vi "Add Device.vi"(8 "error in (no error)":errorcluster, 10 "Device":refnum<class "Hardware.lvclass">, 11 "Controller in":refnum<class "Controller.lvclass">) -> (0 "error out":errorcluster, 3 "Controller out":refnum<class "Controller.lvclass">)   [LabVIEW 2016, in "Controller Actor.lvlib" / "Controller.lvclass"]
uses:
  <userlib>/Common Components/Controller/Controller.lvclass
  C:/Program Files (x86)/National Instruments/LabVIEW 2016/vi.lib/ActorFramework/Actor/Actor.lvclass
  <userlib>/Common Components/Hardware/Abstract Hardware/Hardware.lvclass
  <userlib>/Common Components/Controller/Controller.lvclass/Controller.ctl
  <vilib>/ActorFramework/Actor/Actor.lvclass/Actor.ctl
  <vilib>/ActorFramework/Message Enqueuer/Message Enqueuer.lvclass/Message Enqueuer.ctl
  <vilib>/ActorFramework/Message Enqueuer/Init from Existing Queue.vi
  <vilib>/ActorFramework/Message Enqueuer/Message Enqueuer.lvclass
  <userlib>/Common Components/Controller/Messages/Log Status/Log Status.lvclass
  <vilib>/ActorFramework/Actor/Actor.lvclass
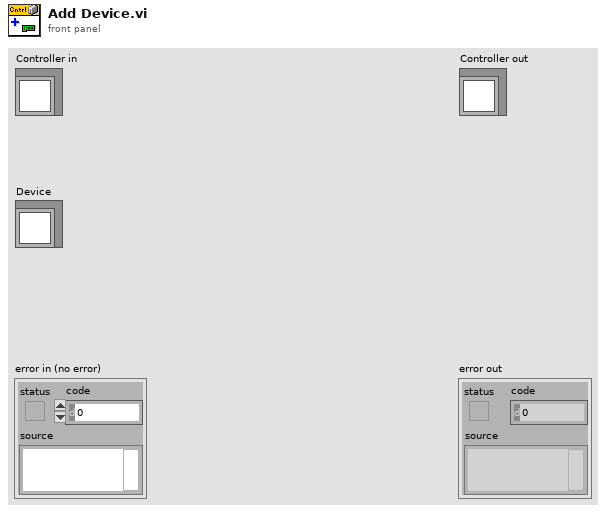
[diagram p1: front panel]
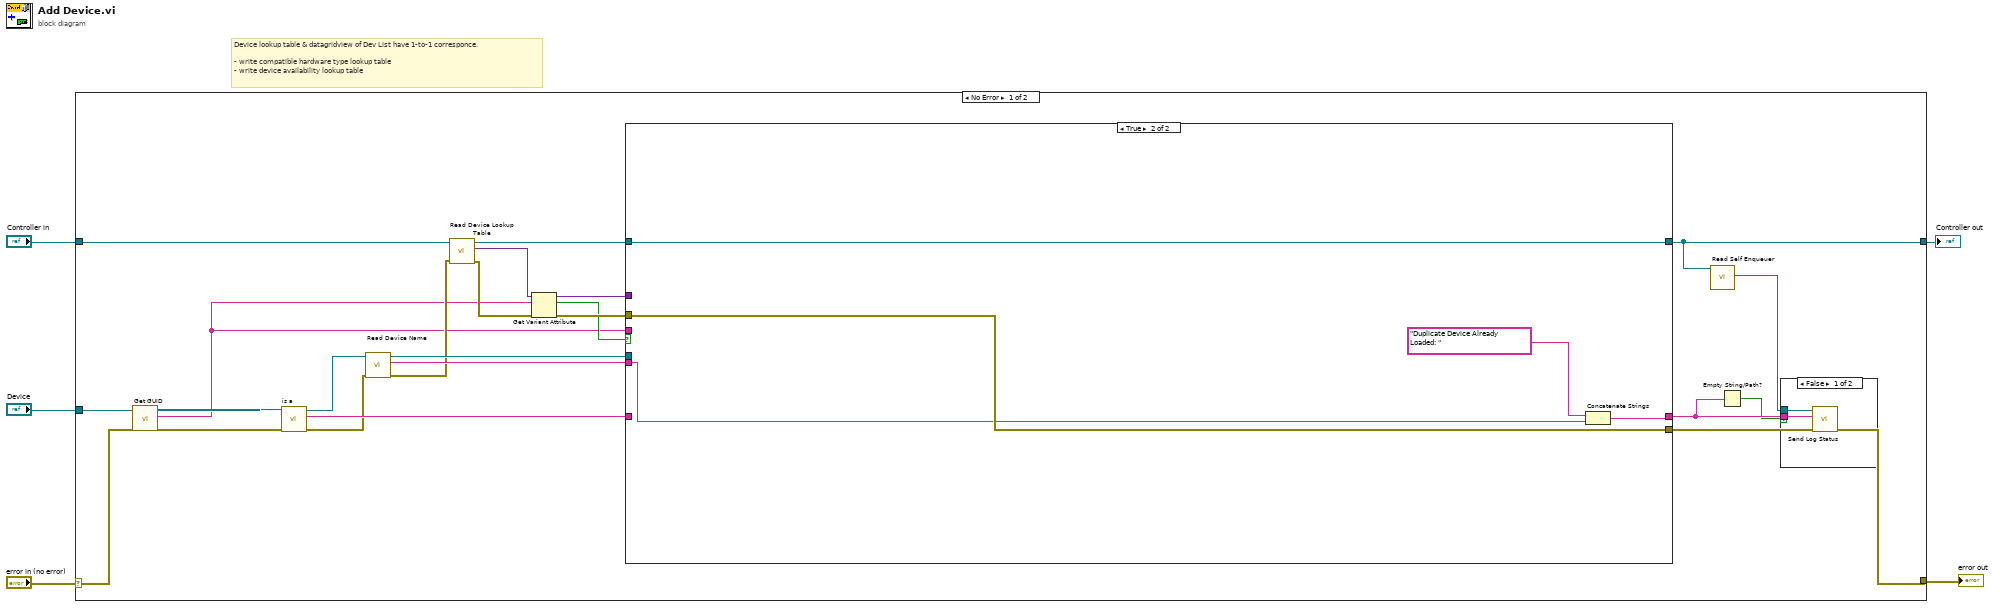
[diagram p0: block diagram]
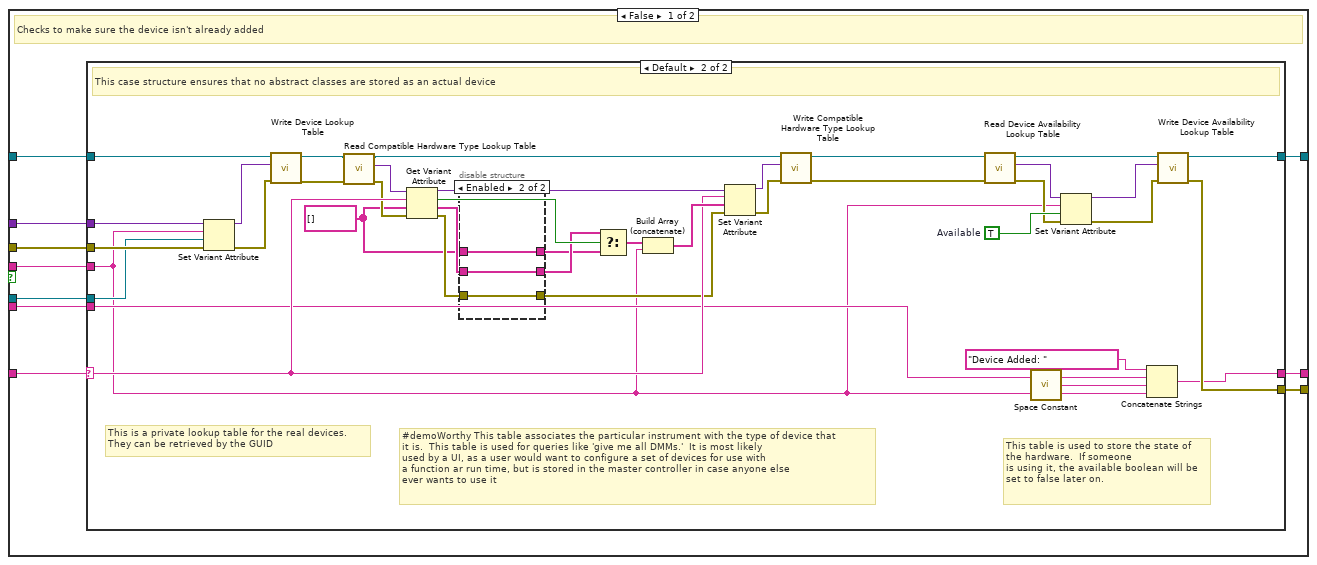
[diagram p3: hidden frame]
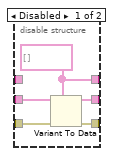
[diagram p5: hidden frame]
diagram:
  # "Device lookup table & datagridview of Dev List have 1-to-1 corresponce.\n\n- write compatible hardware type lookup table\n- write device availability lookup table"
  n1 = case shown="No Error" "error in (no error)" {
    selector: "error in (no error)" -> [w8 w96]
    tunnel: [w27 w96] -> w4
    tunnel: [w19 w95] -> w2
    tunnel: "Controller in" -> [w14 w95]
    tunnel: "Device" -> [w15 _]
    frame No Error {
      n2 = call <userlib>:"Get GUID.vi"("error in (no error)"=w8, "Hardware in"=w15) -> ("error out"=w7:errorcluster, "GUID"=w6:string, "Hardware out"=w9:refnum<class "Hardware.lvclass">)  [unwired: 7 in]
      n3 = call-dynamic "is a.vi"("error in (no error)"=w7, "Hardware in"=w9) -> ("error out"=w24:errorcluster, "is a"=w28:string, "Hardware out"=w25:refnum<class "Hardware.lvclass">)  [unwired: 7 in]
      n4 = call <userlib>:"Read Device Name.vi"("error in (no error)"=w24, "Analog in"=w25) -> ("error out"=w10:errorcluster, "Device Name"=w22:string, "Analog out"=w26:refnum<class "Hardware.lvclass">)  [unwired: 7 in]
      n5 = call <userlib>:"Read Device Lookup Table.vi"("error in (no error)"=w10, "Controller in"=w14) -> ("error out"=w11:errorcluster, "Device Lookup Table (Device GUID -> Device Object)"=w12:variant, "Controller out"=w13:refnum<class "Controller.lvclass">)  [unwired: 7 in]
      n6 = Get Variant Attribute(Variant=w12, name=w6, error in=w11) -> (duplicate Variant=w23:variant, found=w18:bool, error out=w21:errorcluster)  [unwired: 1 in, 1 out]
      n7 = case shown="True" w18 {
        tunnel: w28 -> [w40 _]
        tunnel: [w39 w93] -> w27
        tunnel: w26 -> [w38 _]
        tunnel: w13 -> [w37 w94]
        tunnel: w23 -> [w36 _]
        tunnel: w22 -> [w35 w90]
        tunnel: w21 -> [w34 w93]
        tunnel: [w33 w94] -> w19
        tunnel: [w32 w91] -> w17
        tunnel: w6 -> [w31 _]
        frame False {
          # "Checks to make sure the device isn't already added"
          n8 = case shown="Default" w40 {
            selector: w40 -> [_ w63]
            tunnel: w37 -> [w42 w51]
            tunnel: [w42 w64] -> w33
            tunnel: [w41 w48] -> w39
            tunnel: w38 -> [_ w46]
            tunnel: w35 -> [_ w52]
            tunnel: w36 -> [_ w50]
            tunnel: w34 -> [w41 w49]
            tunnel: [_ w47] -> w32
            tunnel: w31 -> [_ w43]
            frame "Abstract Class" {
            }
            frame Default {
              w44 = string[] []
              w69 = TRUE  # Available
              # "This table is used to store the state of the hardware.  If someone\nis using it, the available boolean will be set to false later on."
              # "This is a private lookup table for the real devices.  \nThey can be retrieved by the GUID"
              # "#demoWorthy This table associates the particular instrument with the type of device that\nit is.  This table is used for queries like 'give me all DMMs.'  It is most likely\nused by a UI, as a user would want to configure a set of devices for use with\na function ar run time, but is stored in the master controller in case anyone else\never wants to use it"
              # "This case structure ensures that no abstract classes are stored as an actual device"
              n9 = Set Variant Attribute(Variant=w50, name=w43, value=w46, error in=w49) -> (Variant out=w81:variant, error out=w60:errorcluster)  [unwired: 1 out]
              n10 = call <userlib>:"Write Device Lookup Table.vi"("error in (no error)"=w60, "Device Lookup Table (Device GUID -> Device Object)"=w81, "Controller in"=w51) -> ("error out"=w61:errorcluster, "Controller out"=w73:refnum<class "Controller.lvclass">)  [unwired: 7 in]
              n11 = call <userlib>:"Read Compatible Hardware Type Lookup Table.vi"("error in (no error)"=w61, "Controller in"=w73) -> ("error out"=w62:errorcluster, "Compatible Hardware Type Lookup Table"=w70:variant, "Controller out"=w72:refnum<class "Controller.lvclass">)  [unwired: 7 in]
              n12 = Get Variant Attribute(Variant=w70, name=w63, default value (empty Variant)=w44, error in=w62) -> (duplicate Variant=w74:variant, found=w78:bool, value=w80:string[], error out=w59:errorcluster)
              n13 = disable-structure shown="Enabled" {
                disable-tunnel: w80 -> [w86 w89]
                disable-tunnel: [w85 w89] -> w76
                disable-tunnel: [w84 w87] -> w75
                disable-tunnel: w59 -> [w83 w88]
                disable-tunnel: [w82 w88] -> w58
                disable-tunnel: w44 -> [_ w87]
                frame Disabled {
                  w84 = string[] []
                  n14 = Variant To Data(error in=w83, type=w84, Variant=w86) -> (data=w85:string[], error out=w82:errorcluster)
                }
                frame Enabled {
                }
              }
              n15 = Select(t=w76, s=w78, f=w75) -> (s? t:f=w77:string[])
              n16 = Build Array (concatenate)(w77, w43) -> (w79:string[])
              n17 = Set Variant Attribute(Variant=w74, name=w63, value=w79, error in=w58) -> (Variant out=w71:variant, error out=w57:errorcluster)  [unwired: 1 out]
              n18 = call <userlib>:"Write Compatible Hardware Type Lookup Table.vi"("error in (no error)"=w57, "Compatible Hardware Type Lookup Table"=w71, "Controller in"=w72) -> ("error out"=w56:errorcluster, "Controller out"=w68:refnum<class "Controller.lvclass">)  [unwired: 7 in]
              n19 = call <userlib>:"Read Device Availability Lookup Table.vi"("error in (no error)"=w56, "Controller in"=w68) -> ("error out"=w55:errorcluster, "Device Availability Lookup Table"=w67:variant, "Controller out"=w65:refnum<class "Controller.lvclass">)  [unwired: 7 in]
              n20 = call <vilib>:"Space Constant.vi"() -> ("String"=w45:string)
              n21 = Set Variant Attribute(Variant=w67, name=w43, value=w69, error in=w55) -> (Variant out=w66:variant, error out=w54:errorcluster)  [unwired: 1 out]
              n22 = Concatenate Strings("Device Added: " ("string"), w52, w45, w43) -> (w47:string)
              n23 = call <userlib>:"Write Device Availability Lookup Table.vi"("error in (no error)"=w54, "Device Availability Lookup Table"=w66, "Controller in"=w65) -> ("error out"=w48:errorcluster, "Controller out"=w64:refnum<class "Controller.lvclass">)  [unwired: 7 in]
            }
          }
        }
        frame True {
          n24 = Concatenate Strings("Duplicate Device Already Loaded: " ("string"), w90) -> (w91:string)
        }
      }
      n25 = call <vilib>:"Read Self Enqueuer.vi"("Actor"=w19) -> ("Self Enqueuer"=w20:refnum<class "Message Enqueuer.lvclass">)  [unwired: 10 in]
      n26 = Empty String/Path?(string/path=w17) -> (empty?=w16:bool)
      n27 = case shown="False" w16 {
        tunnel: w20 -> [w30 _]
        tunnel: w17 -> [w29 _]
        frame False {
          n28 = call <userlib>:"Send Log Status.vi"("String"=w29, "Message Enqueuer in"=w30) -> ()  [unwired: 8 in, 2 out]
        }
        frame True {
        }
      }
    }
    frame Error {
    }
  }
  "error out" <- w4
  "Controller out" <- w2
